vi "Harv_2_9.vi"(0 "HarvSetpoints":dbl[](array[numeric]), 1 "HarvPot":dbl, 3 "Count":i32, 4 "BallAcquired":bool, 5 "FireBallSen":bool, 6 "Fire":bool, 7 "Harvest":bool, 8 "HPButton":bool, 9 "inAuton?":bool, 10 "WinchDown":bool, 11 "AutonMoved":bool, 12 "HarvPivUP":bool, 13 "HarvPivPickupLim":bool) -> (14 "HarvPower":dbl, 15 "HarvRoller":dbl, 16 "AutonReadyToMove":bool, 17 "CountOut":i32, 18 "HarvStart":bool, 19 "HarvCleared":bool)   [LabVIEW 2013]
panel:
  in  "MotorScale":dbl=1.5
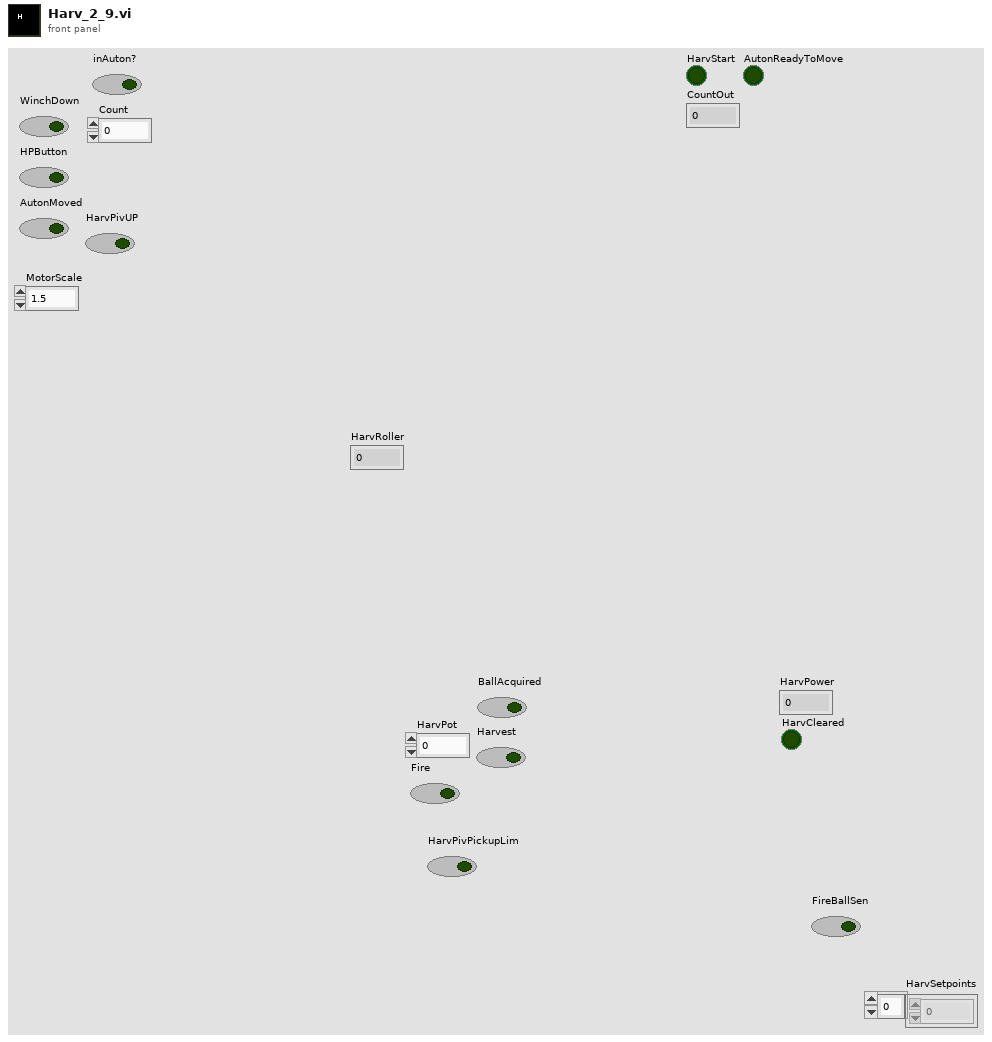
[diagram p1: front panel]
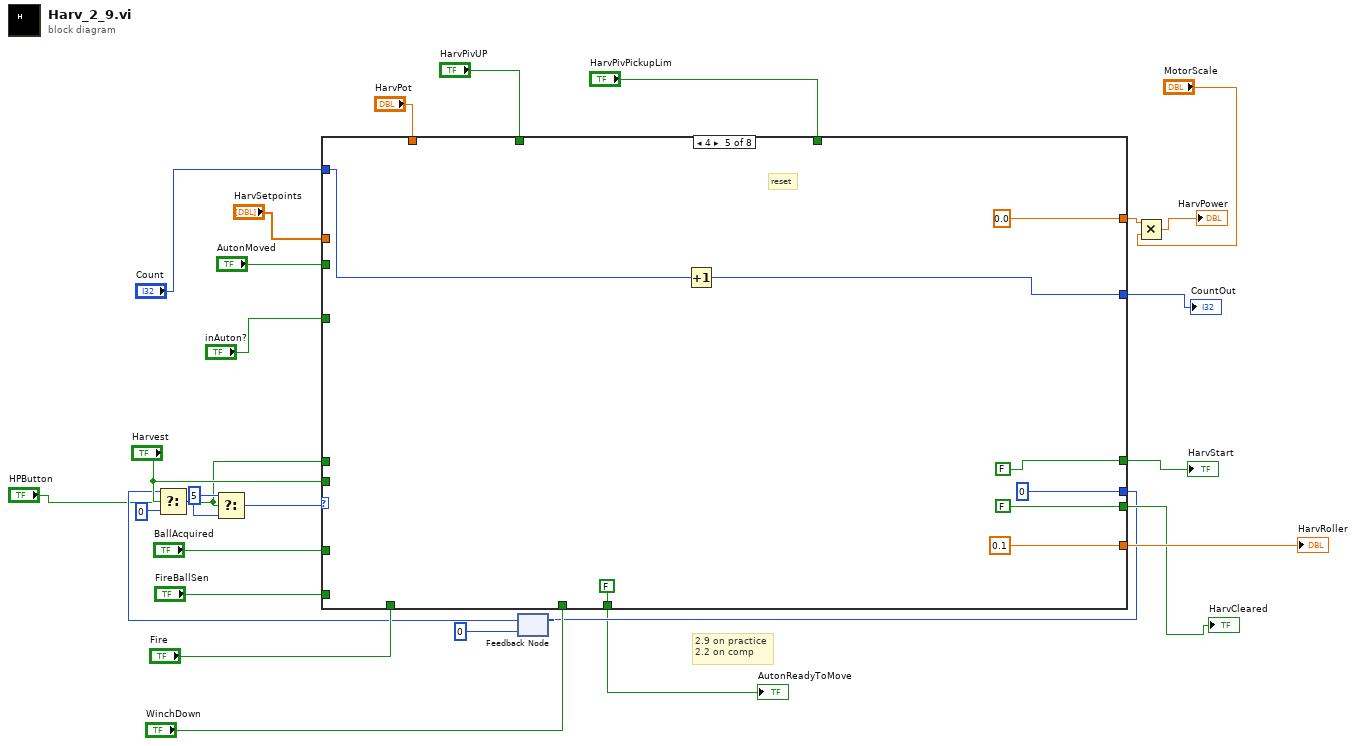
[diagram p0: block diagram]
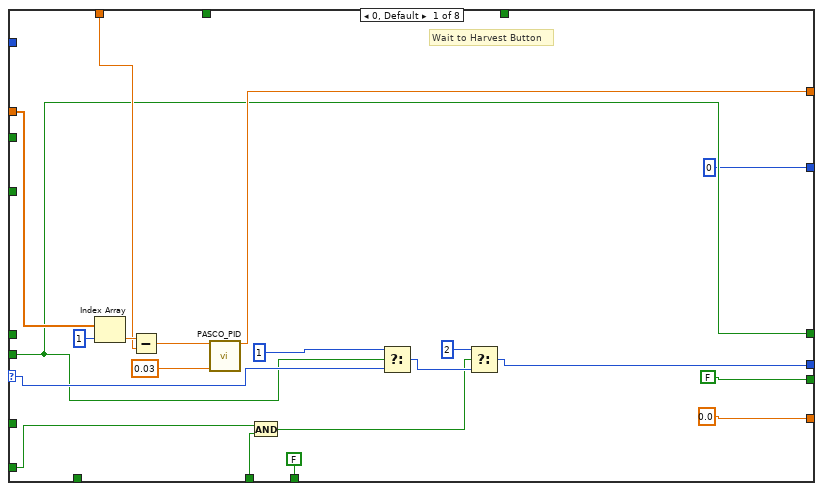
[diagram p2: hidden frame]
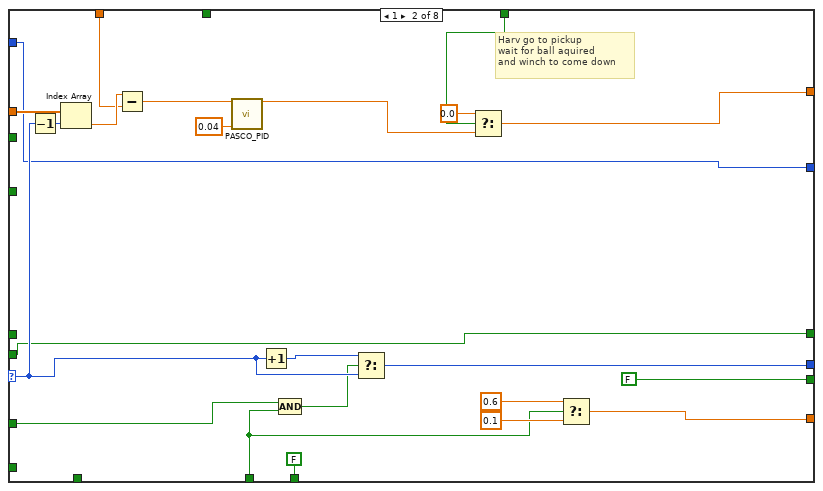
[diagram p3: hidden frame]
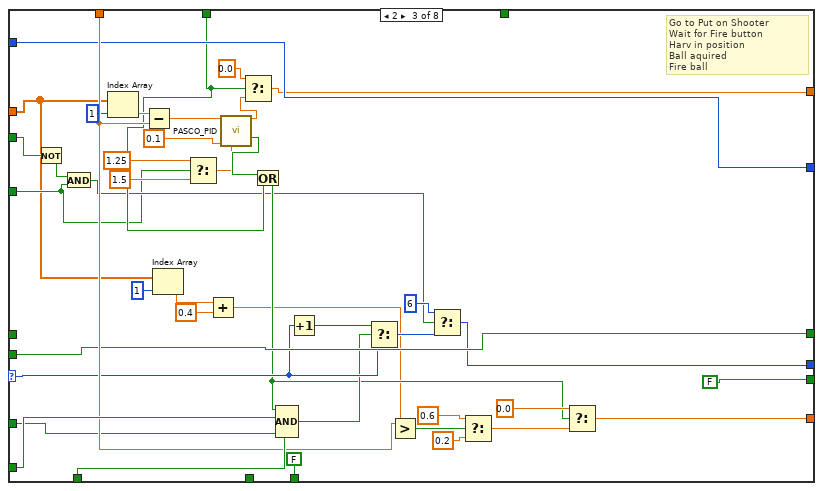
[diagram p4: hidden frame]
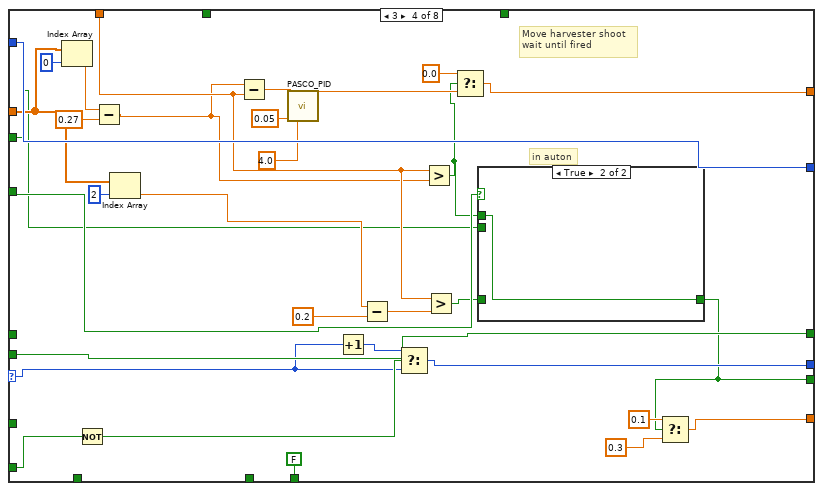
[diagram p5: hidden frame]
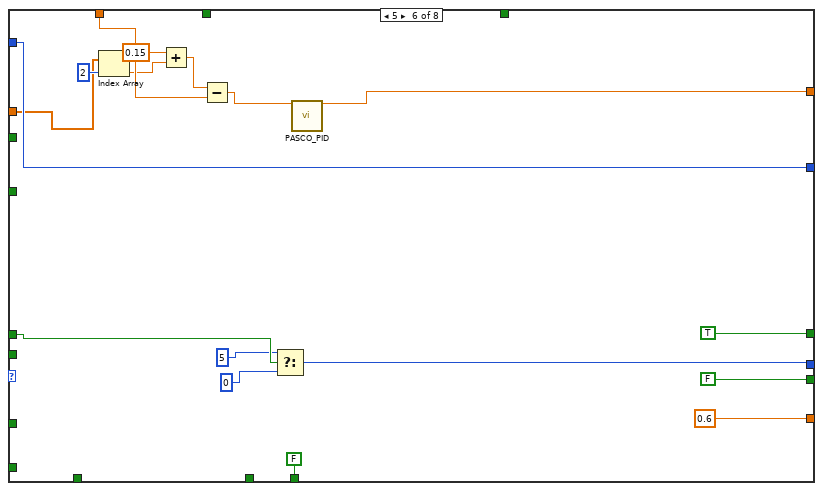
[diagram p7: hidden frame]
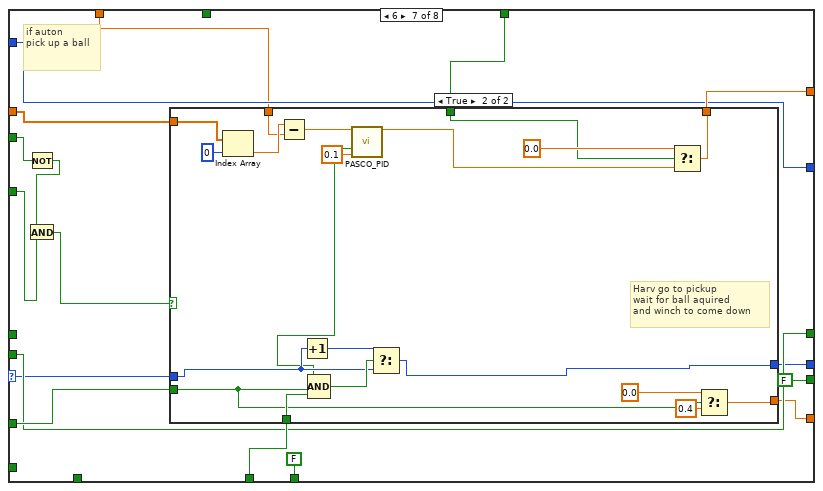
[diagram p8: hidden frame]
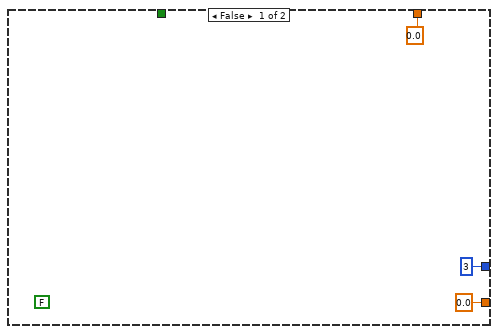
[diagram p9: hidden frame]
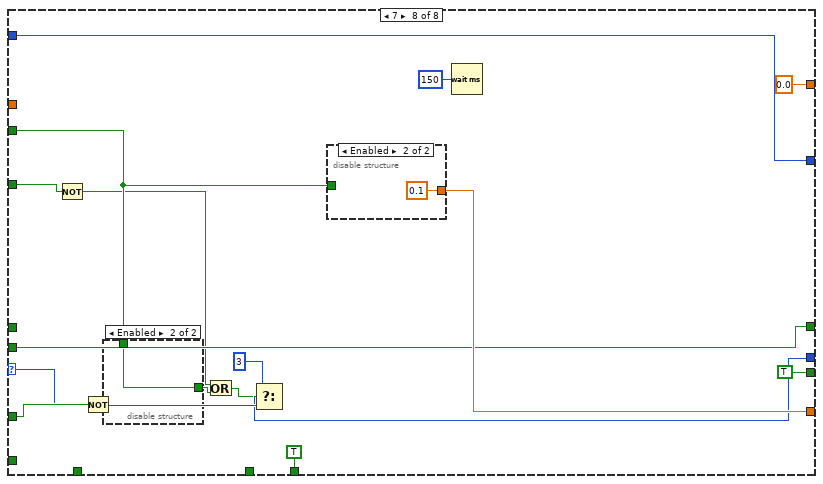
[diagram p10: hidden frame]
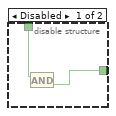
[diagram p11: hidden frame]
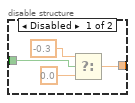
[diagram p12: hidden frame]
diagram:
  # "2.9 on practice\n2.2 on comp"
  n1 = feedback #1(0 ("f")) -> (w21:i32)
  n2 = Select(t=w21, s="Harvest", f=0) -> (s? t:f=w6:i32)
  n3 = Select(t=5, s="HPButton", f=w6) -> (s? t:f=w5:i32)
  n4 = case shown="4" w5 {
    selector: w5 -> [w45 w64 w97 w139 _ _ w181 w222]
    tunnel: "HarvSetpoints" -> [w44 w71 w76 w126 _ w159 w188 _]
    tunnel: "HarvPot" -> [w43 w69 w108 w131 _ w171 w175 _]
    tunnel: [w38 w51 w87 w132 0.0 ("Output") w169 w187 0.0 ("Output")] -> w20
    tunnel: [w35 w66 w89 w144 0 ("t") w164 w182 w221] -> w10
    tunnel: [0.0 ("f") w58 w102 w117 0.1 ("f") 0.6 ("f") w183 w225] -> w26
    tunnel: "BallAcquired" -> [_ w60 w99 _ _ _ w185 w223]
    tunnel: "FireBallSen" -> [w33 _ w111 w142 _ _ _ _]
    tunnel: "Fire" -> [_ _ w110 _ _ _ _ _]
    tunnel: "Harvest" -> [w36 w61 w100 w143 _ _ w184 w224]
    tunnel: [FALSE ("IsThere") FALSE ("IsThere") FALSE ("IsThere") w114 FALSE ("IsThere") FALSE ("IsThere") FALSE ("IsThere") TRUE ("IsThere")] -> w17
    tunnel: "HarvPivPickupLim" -> [_ w53 _ _ _ _ w189 _]
    tunnel: "HarvPivUP" -> [_ _ w92 _ _ _ _ _]
    tunnel: [w36 w61 w100 w143 FALSE ("Harvest") TRUE ("Harvest") w184 w224] -> w14
    tunnel: "WinchDown" -> [w32 w55 _ _ _ _ w186 _]
    tunnel: "inAuton?" -> [_ _ w78 w121 _ _ w176 w214]
    tunnel: [0 ("Count") w54 w96 w138 w150 w168 w180 w227] -> w8
    tunnel: "Count" -> [_ w54 w96 w138 w149 w168 w180 w227]
    tunnel: "HPButton" -> [_ _ _ _ _ w167 _ _]
    tunnel: [FALSE FALSE FALSE FALSE FALSE FALSE FALSE TRUE] -> w2
    tunnel: "AutonMoved" -> [_ _ w84 w118 _ _ w174 w217]
    frame 0, Default {
      # "Wait to Harvest Button"
      n5 = Index Array(array=w44, index=1) -> (element=w46:dbl)
      n6 = Subtract(x=w46, y=w43) -> (x-y=w47:dbl)
      n7 = call "PASCO_PID.vi"("Delta"=w47, "Deadband"=0.03) -> ("Output"=w38:dbl)  [unwired: 12 in, 1 out]
      n8 = And(x=w33, y=w32) -> (x .and. y?=w31:bool)
      n9 = Select(t=1, s=w36, f=w45) -> (s? t:f=w37:i32)
      n10 = Select(t=2, s=w31, f=w37) -> (s? t:f=w35:i32)
    }
    frame 1 {
      # "Harv go to pickup\nwait for ball aquired\nand winch to come down"
      n11 = Decrement(x=w64) -> (x-1=w65:i32)
      n12 = Index Array(array=w71, index=w65) -> (element=w70:dbl)
      n13 = Subtract(x=w70, y=w69) -> (x-y=w68:dbl)
      n14 = call "PASCO_PID.vi"("Delta"=w68, "Deadband"=0.04) -> ("Output"=w52:dbl)  [unwired: 12 in, 1 out]
      n15 = Increment(x=w64) -> (x+1=w67:i32)
      n16 = Compound Arithmetic op=AND(w60, w55) -> (w59:bool)
      n17 = Select(t=w67, s=w59, f=w64) -> (s? t:f=w66:i32)
      n18 = Select(t=0.0, s=w53, f=w52) -> (s? t:f=w51:dbl)
      n19 = Select(t=0.6, s=w55, f=0.1) -> (s? t:f=w58:dbl)
    }
    frame 2 {
      # "Go to Put on Shooter\nWait for Fire button\nHarv in position\nBall aquired \nFire ball"
      n20 = Not(x=w84) -> (.not. x?=w83:bool)
      n21 = And(x=w83, y=w78) -> (x .and. y?=w82:bool)
      n22 = Index Array(array=w76, index=1) -> (element=w113:dbl)
      n23 = Subtract(x=w113, y=w108) -> (x-y=w112:dbl)
      n24 = Index Array(array=w76, index=1) -> (element=w74:dbl)
      n25 = Select(t=1.25, s=w78, f=1.5) -> (s? t:f=w81:dbl)
      n26 = Add(x=w74, y=0.4) -> (x+y=w72:dbl)
      n27 = call "PASCO_PID.vi"("Delta"=w112, "Deadband"=0.1, "P Gain"=w81) -> ("Output"=w95:dbl, "IsThere"=w93:bool)  [unwired: 11 in]
      n28 = Select(t=0.0, s=w92, f=w95) -> (s? t:f=w87:dbl)
      n29 = Or(x=w93, y=w92) -> (x .or. y?=w85:bool)
      n30 = Compound Arithmetic op=AND(w85, w111, w110, w99) -> (w86:bool)
      n31 = Increment(x=w97) -> (x+1=w98:i32)
      n32 = Select(t=w98, s=w86, f=w97) -> (s? t:f=w90:i32)
      n33 = Greater?(x=w108, y=w72) -> (0:w107:bool)
      n34 = Select(t=6, s=w82, f=w90) -> (s? t:f=w89:i32)
      n35 = Select(t=0.6, s=w107, f=0.2) -> (s? t:f=w103:dbl)
      n36 = Select(t=0.0, s=w85, f=w103) -> (s? t:f=w102:dbl)
    }
    frame 3 {
      # "in auton"
      # "Move harvester shoot\nwait until fired"
      n37 = Index Array(array=w126, index=0) -> (element=w125:dbl)
      n38 = Not(x=w142) -> (.not. x?=w141:bool)
      n39 = Subtract(x=w125, y=0.27) -> (x-y=w124:dbl)
      n40 = Index Array(array=w126, index=2) -> (element=w129:dbl)
      n41 = Subtract(x=w124, y=w131) -> (x-y=w137:dbl)
      n42 = call "PASCO_PID.vi"("Delta"=w137, "Deadband"=0.05, "P Gain"=4.0) -> ("Output"=w133:dbl)  [unwired: 11 in, 1 out]
      n43 = Increment(x=w139) -> (x+1=w140:i32)
      n44 = Subtract(x=w129, y=0.2) -> (x-y=w130:dbl)
      n45 = Select(t=w140, s=w141, f=w139) -> (s? t:f=w144:i32)
      n46 = Greater?(x=w131, y=w124) -> (0:w119:bool)
      n47 = Greater?(x=w131, y=w130) -> (0:w120:bool)
      n48 = Select(t=0.0, s=w119, f=w133) -> (s? t:f=w132:dbl)
      n49 = case shown="True" w121 {
        tunnel: [w146 w147] -> w114
        tunnel: w120 -> [w146 _]
        tunnel: w119 -> [_ w147]
        tunnel: w118 -> [_ _]
        frame False {
        }
        frame True {
        }
      }
      n50 = Select(t=0.1, s=w114, f=0.3) -> (s? t:f=w117:dbl)
    }
    frame 4 {
      # "reset"
      n51 = Increment(x=w149) -> (x+1=w150:i32)
    }
    frame 5 {
      n52 = Index Array(array=w159, index=2) -> (element=w157:dbl)
      n53 = Add(x=0.15, y=w157) -> (x+y=w156:dbl)
      n54 = Subtract(x=w156, y=w171) -> (x-y=w170:dbl)
      n55 = Select(t=5 ("index"), s=w167, f=0 ("index")) -> (s? t:f=w164:i32)
      n56 = call "PASCO_PID.vi"("Delta"=w170) -> ("Output"=w169:dbl)  [unwired: 13 in, 1 out]
    }
    frame 6 {
      # "if auton \npick up a ball"
      n57 = Not(x=w174) -> (.not. x?=w173:bool)
      n58 = And(x=w173, y=w176) -> (x .and. y?=w177:bool)
      n59 = case shown="True" w177 {
        tunnel: w189 -> [_ w208]
        tunnel: w188 -> [_ w207]
        tunnel: [0.0 ("Output") w205] -> w187
        tunnel: w186 -> [_ w204]
        tunnel: w185 -> [_ w202]
        tunnel: [0.0 ("f") w203] -> w183
        tunnel: [3 w198] -> w182
        tunnel: w181 -> [_ w196]
        tunnel: w175 -> [_ w194]
        frame False {
          (unwired) FALSE
        }
        frame True {
          # "Harv go to pickup\nwait for ball aquired\nand winch to come down"
          n60 = Index Array(array=w207, index=0) -> (element=w195:dbl)
          n61 = Subtract(x=w195, y=w194) -> (x-y=w209:dbl)
          n62 = Increment(x=w196) -> (x+1=w197:i32)
          n63 = call "PASCO_PID.vi"("Delta"=w209, "Deadband"=0.1) -> ("Output"=w211:dbl, "IsThere"=w193:bool)  [unwired: 12 in]
          n64 = Compound Arithmetic op=AND(w193, w202, w204) -> (w199:bool)
          n65 = Select(t=w197, s=w199, f=w196) -> (s? t:f=w198:i32)
          n66 = Select(t=0.0, s=w208, f=w211) -> (s? t:f=w205:dbl)
          n67 = Select(t=0.0, s=w202, f=0.4) -> (s? t:f=w203:dbl)
        }
      }
    }
    frame 7 {
      n68 = Not(x=w214) -> (.not. x?=w213:bool)
      n69 = Not(x=w223) -> ()  [unwired: 1 out]
      n70 = disable-structure shown="Enabled" {
        disable-tunnel: w217 -> [w231 w232]
        disable-tunnel: [w230 w232] -> w215
        frame Disabled {
          n71 = And(x=w231, y=w230) -> (x .and. y?=w229:bool)
        }
        frame Enabled {
        }
      }
      n72 = Or(x=w213, y=w215) -> (x .or. y?=w216:bool)
      n73 = Select(t=3, s=w216, f=w222) -> (s? t:f=w221:i32)
      n74 = disable-structure shown="Enabled" {
        disable-tunnel: [w236 0.1 ("f")] -> w225
        disable-tunnel: w217 -> [w233 _]
        frame Disabled {
          n75 = Select(t=-0.3, s=w233, f=0.0) -> (s? t:f=w236:dbl)
        }
        frame Enabled {
        }
      }
      n76 = Wait (ms)(milliseconds to wait=u32 150) -> ()  [unwired: 1 out]
    }
  }
  "HarvRoller" <- w26
  "HarvCleared" <- w17
  "HarvStart" <- w14
  "CountOut" <- w8
  "AutonReadyToMove" <- w2
  n77 = feedback-in #1(w10) -> ()
  n78 = Multiply(x=w20, y="MotorScale") -> (x*y=→"HarvPower":dbl)
